vi "Chat.vi"(6 "UserTask":T1, 8 "Error Input":errorcluster, 9 "AgentMessageEventHandler":refnum<k24>, 10 "SessionId":string, 11 "LiteAgentSDK Input":refnum<k24>) -> (0 "Error Output":errorcluster, 3 "LiteAgentSDK Output":refnum<k24>)   [LabVIEW 2017, in "LiteAgentSDK.lvlib"]
uses:
  LiteAgentSDK.lvlib
  C:/Users/Jan/Projects/LiteAgentSDK-LabVIEW/Source/Bin/LiteAgentSDK.LabVIEW.dll
  Bin/LiteAgentSDK.LabVIEW.dll
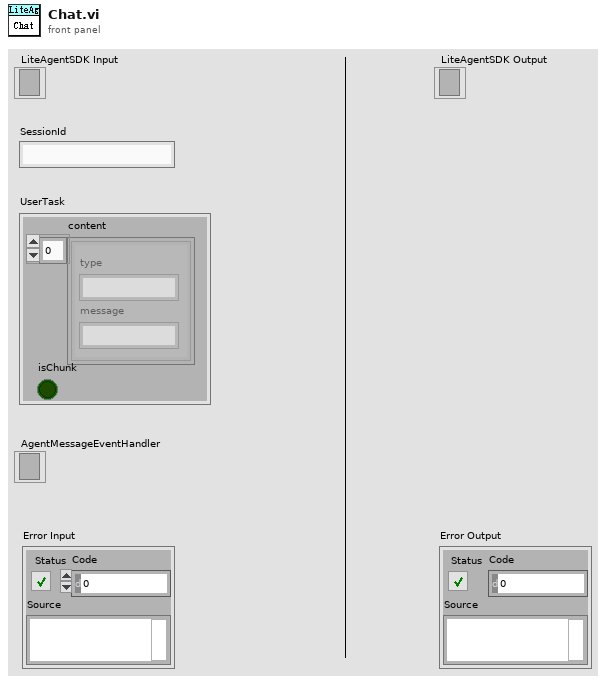
[diagram p1: front panel]
types:
  T1 = cluster{"content":cluster{"type":string, "message":string}[], "isChunk":bool}
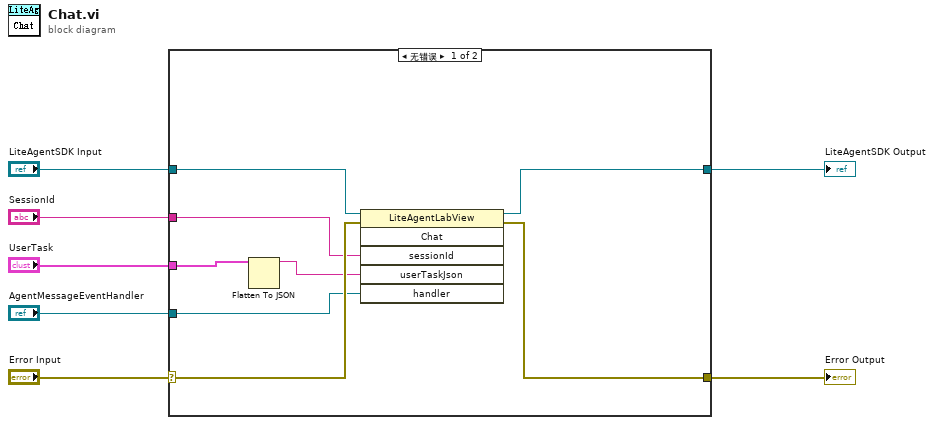
[diagram p0: block diagram]
diagram:
  n1 = case shown="无错误" "Error Input" {
    selector: "Error Input" -> [w15 w16]
    tunnel: "LiteAgentSDK Input" -> [w14 w17]
    tunnel: [w13 w17] -> w2
    tunnel: [w12 w16] -> w6
    tunnel: "SessionId" -> [w11 _]
    tunnel: "UserTask" -> [w10 _]
    tunnel: "AgentMessageEventHandler" -> [w8 _]
    frame No Error {
      n2 = Flatten To JSON(anything=w10) -> (JSON string=w9:string)  [unwired: 2 in, 1 out]
      n3 = invoke on="调用节点" class="LiteAgentLabView" method="Chat"(reference=w14, error in=w15, "sessionId"=w11, "userTaskJson"=w9, "handler"=w8) -> (reference out=w13:refnum<k24>, error out=w12:errorcluster)  [unwired: 1 in, 4 out]
    }
    frame Error {
    }
  }
  "Error Output" <- w6
  "LiteAgentSDK Output" <- w2
